vi "findChannelByName.vi"(8 "error in (no error)":errorcluster, 10 "channel_name":string, 11 "DeviceArray in":refnum<class "DeviceArray.lvclass">) -> (0 "error out":errorcluster, 1 "Channel.lvclass":refnum<class "Channel.lvclass">, 2 "device.lvclass":refnum<class "device.lvclass">, 3 "DeviceArray out":refnum<class "DeviceArray.lvclass">, 4 "found?":bool)   [LabVIEW 2011, in "Tools.lvlib" / "DatabaseHelpers.lvlib" / "DeviceArray.lvclass"]
uses:
  DeviceArray.lvclass
  Channel/Channel.lvclass
  device/device.lvclass
  DeviceArray.lvclass/DeviceArray.ctl
  ChannelArray/ChannelArray.lvclass
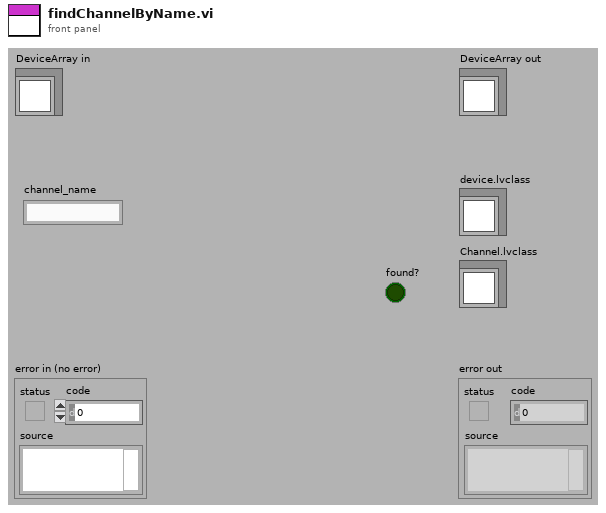
[diagram p1: front panel]
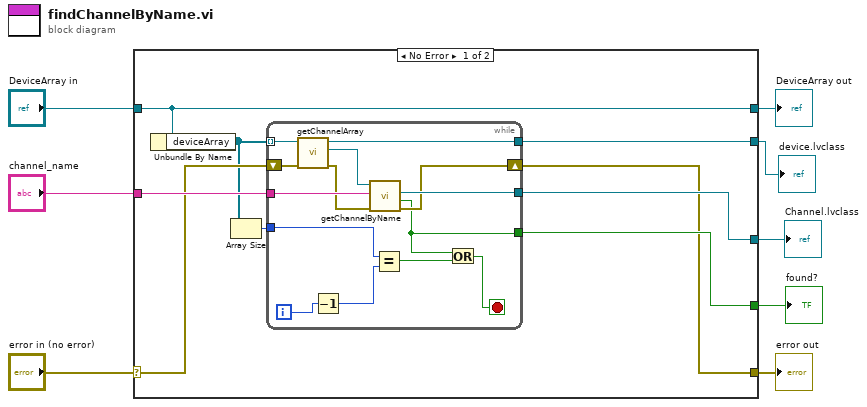
[diagram p0: block diagram]
diagram:
  n1 = case shown="No Error" "error in (no error)" {
    selector: "error in (no error)" -> [w15 w33]
    tunnel: [w9 w33] -> w7
    tunnel: [w17 w32] -> w5
    tunnel: "DeviceArray in" -> [w17 w32]
    tunnel: "channel_name" -> [w16 _]
    tunnel: [w12 _] -> w3
    tunnel: [w11 _] -> w2
    tunnel: [w10 _] -> w1
    frame No Error {
      n2 = Unbundle By Name(w17) -> ("deviceArray"=w14:refnum<class "device.lvclass">[])
      n3 = Array Size(array=w14) -> (size(s)=w13:i32)
      n4 = while {
        tunnel: w14 -> [w31] mode=indexing
        tunnel: w16 -> [w29]
        shift-right: [w24] -> w9
        shift-left: w15 -> [w27]
        tunnel: [w26] -> w10
        tunnel: [w25] -> w11
        tunnel: w13 -> [w22]
        tunnel: [w18] -> w12
        i -> [w23]
        stop <- w19 stop-if-true
        n5 = call "getChannelArray.vi"("error in (no error)"=w27, "device.lvclass in"=w31) -> ("error out"=w28:errorcluster, "ChannelArray.lvclass"=w30:refnum<class "ChannelArray.lvclass">, "device.lvclass out"=w25:refnum<class "device.lvclass">)  [unwired: 7 in]
        n6 = Decrement(x=w23) -> (x-1=w21:i32)
        n7 = call-dynamic "getChannelByName.vi"("error in (no error)"=w28, "channel_name"=w29, "ChannelArray in"=w30) -> ("error out"=w24:errorcluster, "found?"=w18:bool, "Channel"=w26:refnum<class "Channel.lvclass">)  [unwired: 5 in, 1 out]
        n8 = Equal?(x=w22, y=w21) -> (x = y?=w20:bool)
        n9 = Or(x=w18, y=w20) -> (x .or. y?=w19:bool)
      }
    }
    frame Error {
    }
  }
  "error out" <- w7
  "DeviceArray out" <- w5
  "Channel.lvclass" <- w1
  "device.lvclass" <- w2
  "found?" <- w3
